vi "QD_UPS.vi"(0 "State_and_Data_In":T1, 1 "Max_Queue_Size_In":i32=-1, 2 "Queue_Name_In":string, 5 "State_and_Data_N_In":T1[](array[typedef]), 7 "Time_Out_In_ms (-1)":i32, 11 "Error_In":errorcluster, 13 "Queue_Operation":T2=enum."Flush") -> (4 "State_and_Data_Out":T1, 15 "Error_Out":errorcluster)   [LabVIEW 2021]
doc: "Used to transfer data from one vi to another using queue."
uses:
  Controls/State_and_Data.ctl
  Controls/Error_Data.ctl
  Controls/Queue_Operation_Select.ctl
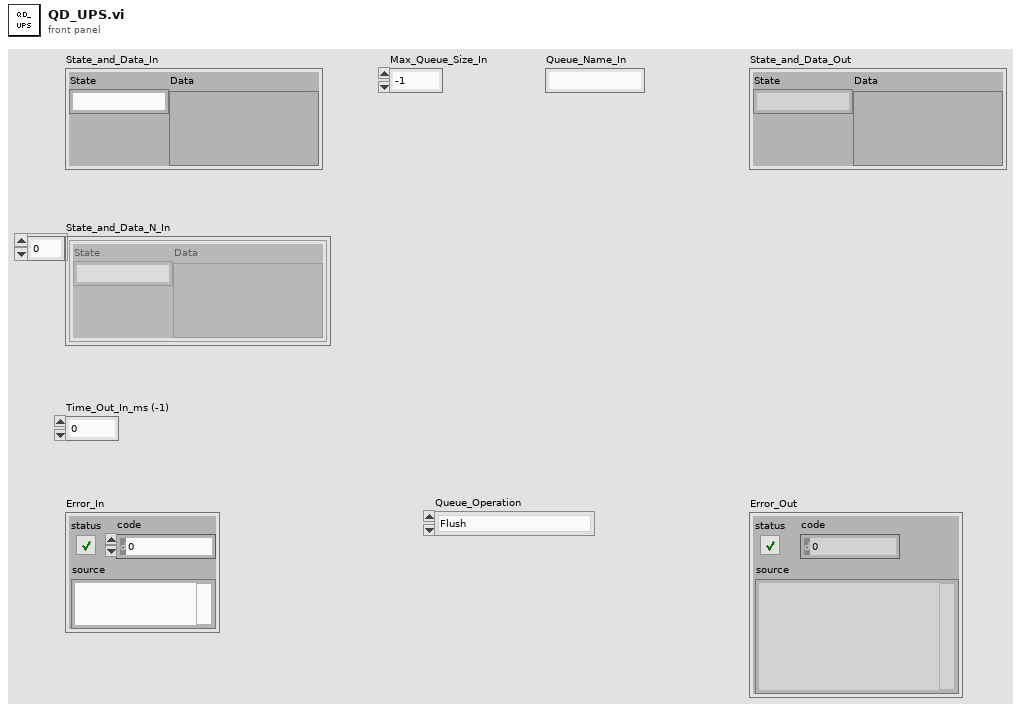
[diagram p1: front panel]
types:
  T1 = typedef "State_and_Data.ctl" = cluster{"State":string, "Data":variant}
  T2 = typedef "Queue_Operation_Select.ctl" = enum16{"Obtain_Queue", "Enqueue", "Enqueue_First", "Enqueue_N", "Lossy_Enqueue", "Preview", "Queue_Status", "Dequeue", "Flush", "Release_Queue"}
  T3 = typedef "Error_Data.ctl" = cluster{"Module_Name":string, "Error":errorcluster}
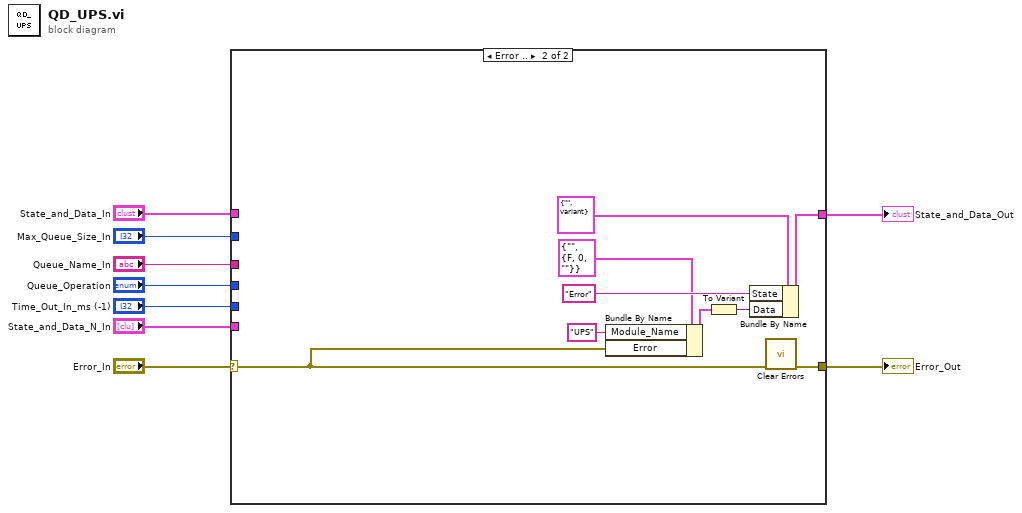
[diagram p0: block diagram]
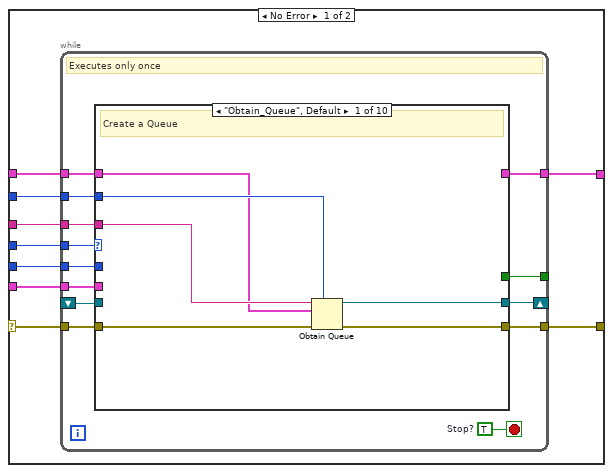
[diagram p2: hidden frame]
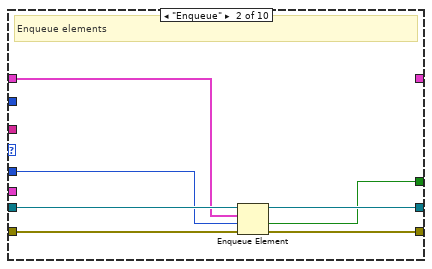
[diagram p3: hidden frame]
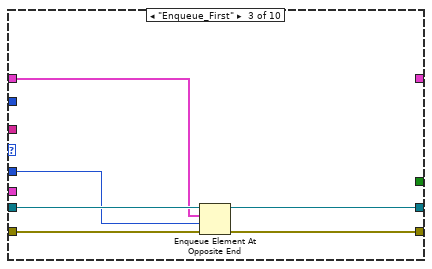
[diagram p4: hidden frame]
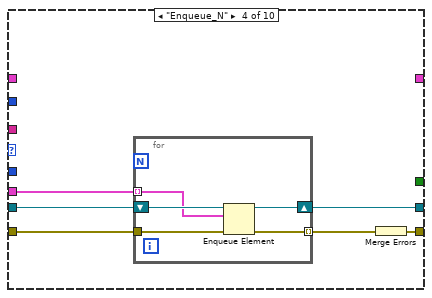
[diagram p5: hidden frame]
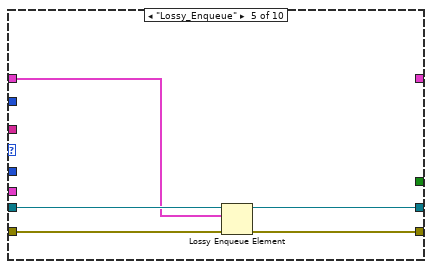
[diagram p6: hidden frame]
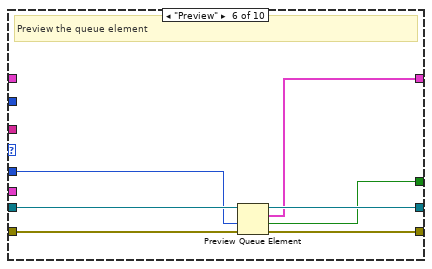
[diagram p7: hidden frame]
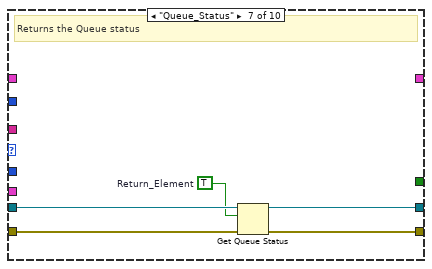
[diagram p8: hidden frame]
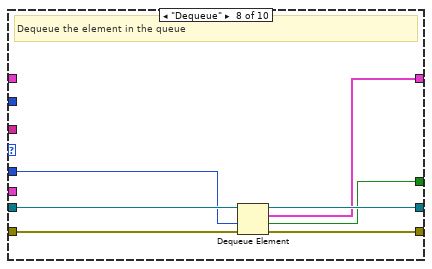
[diagram p9: hidden frame]
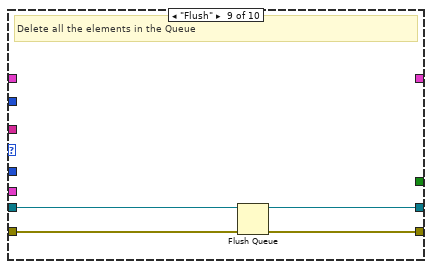
[diagram p10: hidden frame]
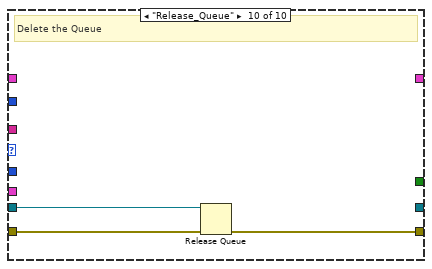
[diagram p11: hidden frame]
diagram:
  n1 = case shown="Error .." "Error_In" {
    selector: "Error_In" -> [w10 w95]
    tunnel: "Max_Queue_Size_In" -> [w18 _]
    tunnel: [w17 w93] -> w8
    tunnel: "Time_Out_In_ms (-1)" -> [w16 _]
    tunnel: "Queue_Operation" -> [w15 _]
    tunnel: "Queue_Name_In" -> [w14 _]
    tunnel: "State_and_Data_In" -> [w13 _]
    tunnel: [w12 w100] -> w3
    tunnel: "State_and_Data_N_In" -> [w11 _]
    frame No Error {
      n2 = while {
        tunnel: w18 -> [w31]
        tunnel: w16 -> [w28]
        tunnel: w15 -> [w25]
        shift-right: [w26] -> _
        shift-left: _ -> [w22]
        tunnel: w13 -> [w29]
        tunnel: [w27] -> w12
        tunnel: w14 -> [w24]
        tunnel: w10 -> [w23]
        tunnel: [w30] -> w17
        tunnel: [w20] -> _
        tunnel: w11 -> [w19]
        stop <- w21 stop-if-true
        w21 = TRUE  # Stop?
        # "Executes only once"
        n3 = case shown="\"Obtain_Queue\", Default" w25 {
          tunnel: w23 -> [w37 w44 w50 w56 w65 w72 w77 w84 w88 w92]
          tunnel: w24 -> [w35 _ _ _ _ _ _ _ _ _]
          tunnel: w31 -> [w34 _ _ _ _ _ _ _ _ _]
          tunnel: [w32 w40 w45 w53 w64 w71 w76 w83 w87 _] -> w26
          tunnel: [w36 w43 w49 w51 w63 w70 w75 w81 w86 w91] -> w30
          tunnel: w22 -> [_ w42 w48 w54 w66 w73 w78 w85 w89 w90]
          tunnel: w29 -> [w33 w41 w47 _ w62 _ _ _ _ _]
          tunnel: w28 -> [_ w39 w46 _ _ w69 _ w80 _ _]
          tunnel: [_ _ _ _ _ w68 _ w82 _ _] -> w27
          tunnel: [_ w38 _ _ _ w67 _ w79 _ _] -> w20
          tunnel: w19 -> [_ _ _ w52 _ _ _ _ _ _]
          frame "Obtain_Queue", Default {
            # "Create a Queue"
            n4 = Obtain Queue(max queue size (-1, unlimited)=w34, name (unnamed)=w35, element data type=w33, error in (no error)=w37) -> (queue out=w32:refnum<queue>, error out=w36:errorcluster)  [unwired: 1 in, 1 out]
          }
          frame "Enqueue" {
            # "Enqueue elements"
            n5 = Enqueue Element(queue=w42, element=w41, timeout in ms (-1)=w39, error in (no error)=w44) -> (queue out=w40:refnum<queue>, timed out?=w38:bool, error out=w43:errorcluster)
          }
          frame "Enqueue_First" {
            n6 = Enqueue Element At Opposite End(queue=w48, element=w47, timeout in ms (-1)=w46, error in (no error)=w50) -> (queue out=w45:refnum<queue>, error out=w49:errorcluster)  [unwired: 1 out]
          }
          frame "Enqueue_N" {
            n7 = for {
              tunnel: w52 -> [w57] mode=indexing
              tunnel: w56 -> [w61]
              tunnel: [w60] -> w55 mode=indexing
              shift-right: [w58] -> w53
              shift-left: w54 -> [w59]
              n8 = Enqueue Element(queue=w59, element=w57, error in (no error)=w61) -> (queue out=w58:refnum<queue>, error out=w60:errorcluster)  [unwired: 1 in, 1 out]
            }
            n9 = Merge Errors(w55) -> (w51:errorcluster)
          }
          frame "Lossy_Enqueue" {
            n10 = Lossy Enqueue Element(queue=w66, element=w62, error in (no error)=w65) -> (queue out=w64:refnum<queue>, error out=w63:errorcluster)  [unwired: 2 out]
          }
          frame "Preview" {
            # "Preview the queue element"
            n11 = Preview Queue Element(queue=w73, timeout in ms (-1)=w69, error in (no error)=w72) -> (queue out=w71:refnum<queue>, element=w68:T1, timed out?=w67:bool, error out=w70:errorcluster)
          }
          frame "Queue_Status" {
            w74 = TRUE  # Return_Element
            # "Returns the Queue status"
            n12 = Get Queue Status(queue=w78, return elements? (F)=w74, error in (no error)=w77) -> (queue out=w76:refnum<queue>, error out=w75:errorcluster)  [unwired: 6 out]
          }
          frame "Dequeue" {
            # "Dequeue the element in the queue"
            n13 = Dequeue Element(queue=w85, timeout in ms (-1)=w80, error in (no error)=w84) -> (queue out=w83:refnum<queue>, element=w82:T1, timed out?=w79:bool, error out=w81:errorcluster)
          }
          frame "Flush" {
            # "Delete all the elements in the Queue"
            n14 = Flush Queue(queue=w89, error in (no error)=w88) -> (queue out=w87:refnum<queue>, error out=w86:errorcluster)  [unwired: 1 out]
          }
          frame "Release_Queue" {
            # "Delete the Queue"
            n15 = Release Queue(queue=w90, error in (no error)=w92) -> (error out=w91:errorcluster)  [unwired: 1 in, 2 out]
          }
        }
      }
    }
    frame Error {
      n16 = Bundle By Name(cluster=T3 {"Module_Name"="", "Error"={"status"=FALSE, "code"=0, "source"=""}} ("Error_Data"), "Module_Name"="UPS", "Error"=w95) -> (w97:T3)
      n17 = To Variant(anything=w97) -> (Variant=w96:variant)
      n18 = Bundle By Name(cluster=T1 {"State"="", "Data"=variant} ("State_and_Data_In"), "State"="Error", "Data"=w96) -> (w100:T1)
      n19 = call <vilib>:"Clear Errors.vi"("error in (no error)"=w95) -> ("error out"=w93:errorcluster)  [unwired: 5 in, 1 out]
    }
  }
  "Error_Out" <- w8
  "State_and_Data_Out" <- w3
